vi "rx_ceEq.vi"(2 "preamble":cdb[](array[numeric])=[-0.7071067811865475+0.7071067811865476i, 0.7071067811865476+0.7071067811865475i, 0.7071067811865474-0.7071067811865477i, 0.7071067811865476+0.7071067811865475i, -0.7071067811865475+0.7071067811865476i, -0.7071067811865477-0.7071067811865475i, 0.7071067811865476+0.7071067811865475i, -0.7071067811865477-0.7071067811865475i, -0.7071067811865475+0.7071067811865476i, 0.7071067811865476+0.7071067811865475i, 0.7071067811865474-0.7071067811865477i, 0.7071067811865476+0.7071067811865475i, -0.7071067811865475+0.7071067811865476i, -0.7071067811865477-0.7071067811865475i, 0.7071067811865476+0.7071067811865475i, -0.7071067811865477-0.7071067811865475i, -0.7071067811865475+0.7071067811865476i, 0.7071067811865476+0.7071067811865475i, 0.7071067811865474-0.7071067811865477i, 0.7071067811865476+0.7071067811865475i, -0.7071067811865475+0.7071067811865476i, -0.7071067811865477-0.7071067811865475i, 0.7071067811865476+0.7071067811865475i, -0.7071067811865477-0.7071067811865475i, -0.7071067811865475+0.7071067811865476i, 0.7071067811865476+0.7071067811865475i, 0.7071067811865474-0.7071067811865477i, 0.7071067811865476+0.7071067811865475i, -0.7071067811865475+0.7071067811865476i, -0.7071067811865477-0.7071067811865475i, 0.7071067811865476+0.7071067811865475i, -0.7071067811865477-0.7071067811865475i, -0.7071067811865475+0.7071067811865476i, 0.7071067811865476+0.7071067811865475i, 0.7071067811865474-0.7071067811865477i, 0.7071067811865476+0.7071067811865475i, -0.7071067811865475+0.7071067811865476i, -0.7071067811865477-0.7071067811865475i, 0.7071067811865476+0.7071067811865475i, -0.7071067811865477-0.7071067811865475i, -0.7071067811865475+0.7071067811865476i, 0.7071067811865476+0.7071067811865475i, 0.7071067811865474-0.7071067811865477i, 0.7071067811865476+0.7071067811865475i, -0.7071067811865475+0.7071067811865476i, -0.7071067811865477-0.7071067811865475i, 0.7071067811865476+0.7071067811865475i, -0.7071067811865477-0.7071067811865475i, -0.7071067811865475+0.7071067811865476i, 0.7071067811865476+0.7071067811865475i, 0.7071067811865474-0.7071067811865477i, 0.7071067811865476+0.7071067811865475i, -0.7071067811865475+0.7071067811865476i, -0.7071067811865477-0.7071067811865475i, 0.7071067811865476+0.7071067811865475i, -0.7071067811865477-0.7071067811865475i, -0.7071067811865475+0.7071067811865476i, 0.7071067811865476+0.7071067811865475i, 0.7071067811865474-0.7071067811865477i, 0.7071067811865476+0.7071067811865475i, -0.7071067811865475+0.7071067811865476i, -0.7071067811865477-0.7071067811865475i, 0.7071067811865476+0.7071067811865475i, -0.7071067811865477-0.7071067811865475i], 3 "symbols":cdb[](array[numeric])) -> (0 "valid?":bool, 1 "eq symbols":cdb[](array[numeric]))   [LabVIEW 2014]
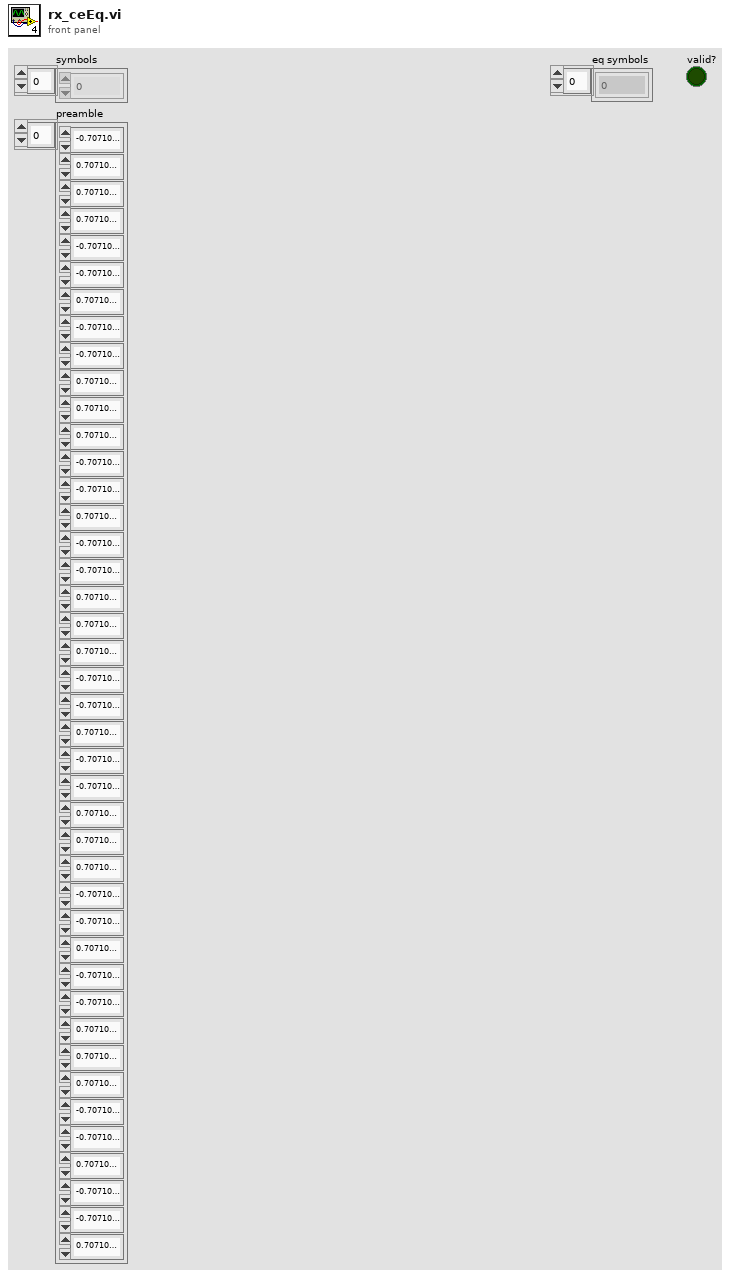
[diagram p1: front panel]
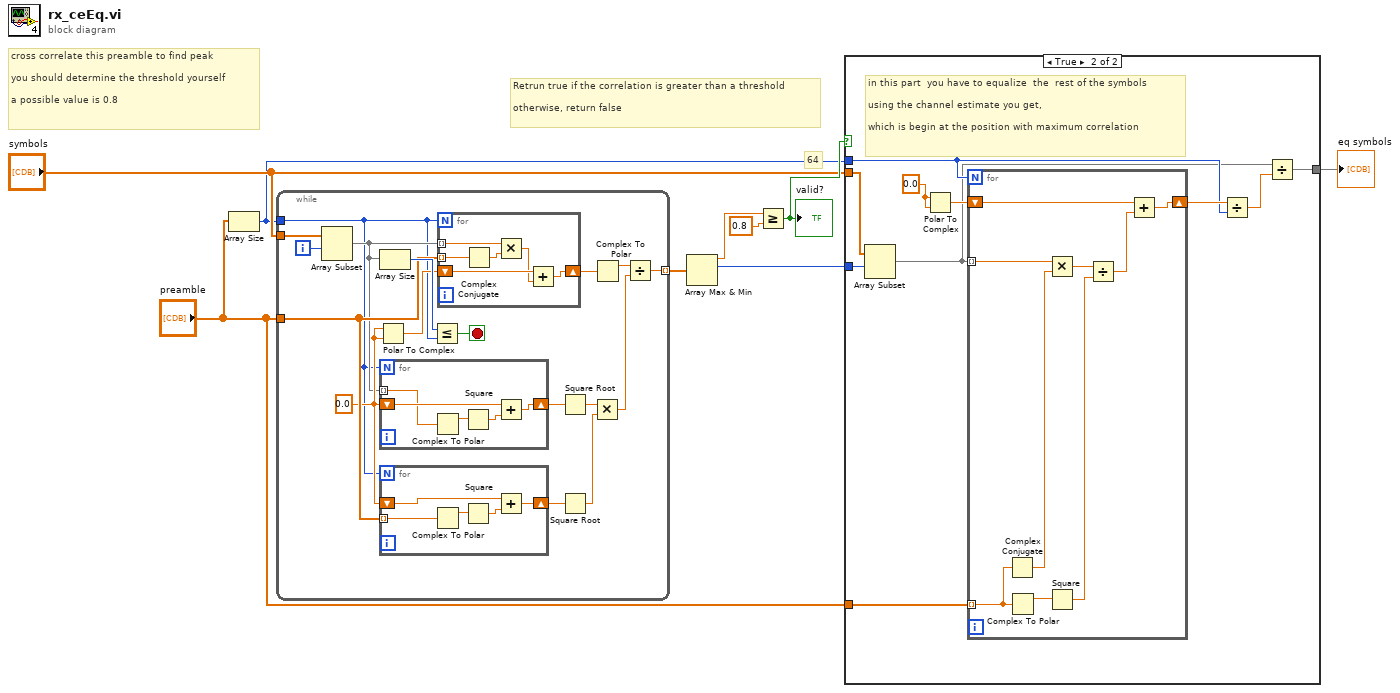
[diagram p0: block diagram]
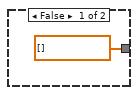
[diagram p2: hidden frame]
diagram:
  # "Retrun true if the correlation is greater than a threshold\n\notherwise, return false"
  # "cross correlate this preamble to find peak \n\nyou should determine the threshold yourself\n\na possible value is 0.8"
  # "64"
  n1 = Array Size(array="preamble") -> (size(s)=w4:i32)
  n2 = while {
    tunnel: "symbols" -> [w26]
    tunnel: w4 -> [w11]
    tunnel: "preamble" -> [w23]
    tunnel: [w10] -> w3 mode=indexing
    i -> [w18]
    stop <- w24 stop-if-true
    w16 = 0.0
    n3 = Array Subset(array=w26, index=w18) -> (w12:cdb[])  [unwired: 1 in]
    n4 = Polar To Complex(1:w16, 2:w16) -> (0:w15:cdb)
    n5 = Array Size(array=w12) -> (size(s)=w25:i32)
    n6 = for {
      N: w11 -> [_]
      tunnel: w12 -> [w34] mode=indexing
      shift-right: [w35] -> w22
      shift-left: w16 -> [w36]
      n7 = Complex To Polar(r * e^(i*theta)=w34) -> (r=w33:dbl)  [unwired: 1 out]
      n8 = Square(x=w33) -> (x^2=w32:dbl)
      n9 = Add(x=w36, y=w32) -> (x+y=w35:dbl)
    }
    n10 = for {
      N: w11 -> [_]
      tunnel: w23 -> [w29] mode=indexing
      shift-right: [w30] -> w21
      shift-left: w16 -> [w31]
      n11 = Complex To Polar(r * e^(i*theta)=w29) -> (r=w28:dbl)  [unwired: 1 out]
      n12 = Square(x=w28) -> (x^2=w27:dbl)
      n13 = Add(x=w31, y=w27) -> (x+y=w30:dbl)
    }
    n14 = Less Or Equal?(x=w25, y=w11) -> (x <= y?=w24:bool)
    n15 = for {
      N: w11 -> [_]
      tunnel: w12 -> [w40] mode=indexing
      tunnel: w23 -> [w42] mode=indexing
      shift-right: [w38] -> w14
      shift-left: w15 -> [w39]
      n16 = Complex Conjugate(1:w42) -> (0:w41:cdb)
      n17 = Multiply(x=w40, y=w41) -> (x*y=w37:cdb)
      n18 = Add(x=w39, y=w37) -> (x+y=w38:cdb)
    }
    n19 = Square Root(x=w22) -> (sqrt(x)=w20:dbl)
    n20 = Square Root(x=w21) -> (sqrt(x)=w19:dbl)
    n21 = Multiply(x=w20, y=w19) -> (x*y=w17:dbl)
    n22 = Complex To Polar(r * e^(i*theta)=w14) -> (r=w13:dbl)  [unwired: 1 out]
    n23 = Divide(x=w13, y=w17) -> (x/y=w10:dbl)
  }
  n24 = Array Max & Min(array=w3) -> (max value=w2:dbl, max index (indices)=w1:i32)  [unwired: 2 out]
  n25 = Greater Or Equal?(x=w2, y=0.8) -> (x >= y?=w7:bool)
  "valid?" <- w7
  n26 = case shown="True" w7 {
    tunnel: [cdb[] [] w44] -> w9
    tunnel: "symbols" -> [_ w53]
    tunnel: "preamble" -> [_ w51]
    tunnel: w1 -> [_ w52]
    tunnel: w4 -> [_ w47]
    frame False {
    }
    frame True {
      w50 = 0.0
      # "in this part  you have to equalize  the  rest of the symbols\n\nusing the channel estimate you get, \n\nwhich is begin at the position with maximum correlation"
      n27 = Array Subset(array=w53, index=w52) -> (w46:cdb[])  [unwired: 1 in]
      n28 = Polar To Complex(1:w50, 2:w50) -> (0:w49:cdb)
      n29 = for {
        N: w47 -> [_]
        tunnel: w46 -> [w61] mode=indexing
        tunnel: w51 -> [w60] mode=indexing
        shift-right: [w54] -> w48
        shift-left: w49 -> [w56]
        n30 = Complex Conjugate(1:w60) -> (0:w62:cdb)
        n31 = Complex To Polar(r * e^(i*theta)=w60) -> (r=w59:dbl)  [unwired: 1 out]
        n32 = Multiply(x=w61, y=w62) -> (x*y=w58:cdb)
        n33 = Square(x=w59) -> (x^2=w57:dbl)
        n34 = Divide(x=w58, y=w57) -> (x/y=w55:cdb)
        n35 = Add(x=w56, y=w55) -> (x+y=w54:cdb)
      }
      n36 = Divide(x=w48, y=w47) -> (x/y=w45:cdb)
      n37 = Divide(x=w46, y=w45) -> (x/y=w44:cdb[])
    }
  }
  "eq symbols" <- w9
